vi "HdrLinePar.vi"(0 "String":string) -> (1 "Paramètre":string, 2 "Valeur":string, 3 "Commentaire":string)   [LabVIEW 2011]
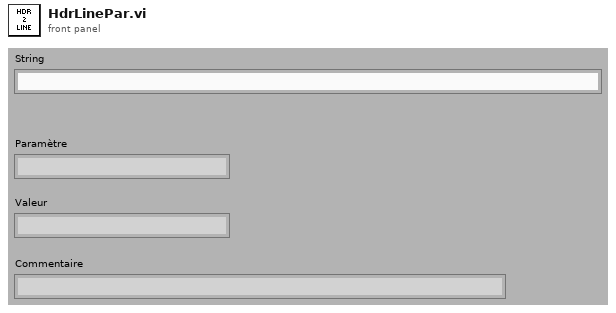
[diagram p1: front panel]
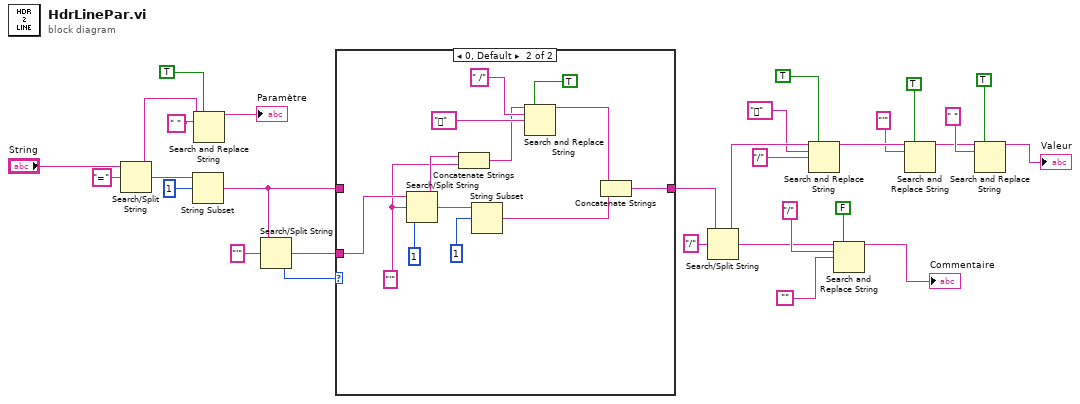
[diagram p0: block diagram]
diagram:
  n1 = Search/Split String(string="String", search string/char (-)="=") -> (substring before match=w25:string, match + rest of string=w27:string)  [unwired: 1 in, 1 out]
  n2 = String Subset(string=w27, offset (0)=1) -> (substring=w18:string)  [unwired: 1 in]
  n3 = Search and Replace String(replace all?=TRUE ("replace all? (F)"), input string=w25, search string=" ") -> (result string=→"Paramètre":string)  [unwired: 5 in, 3 out]
  n4 = Search/Split String(string=w18, search string/char (-)="'") -> (match + rest of string=w17:string, offset of match=w20:i32)  [unwired: 1 in, 1 out]
  n5 = case shown="0, Default" w20 {
    tunnel: [w31 w34] -> w19
    tunnel: w18 -> [w31 _]
    tunnel: w17 -> [_ w44]
    frame -1 {
    }
    frame 0, Default {
      w38 = "'" ("search string/char (-)")
      n6 = Search/Split String(string=w44, search string/char (-)=w38, offset (0)=1) -> (substring before match=w39:string, match + rest of string=w43:string)  [unwired: 1 out]
      n7 = Concatenate Strings(w39, w38) -> (w37:string)
      n8 = String Subset(string=w43, offset (0)=1) -> (substring=w35:string)  [unwired: 1 in]
      n9 = Search and Replace String(replace all?=TRUE ("replace all? (F)"), input string=w37, search string=" /", replace string="" ("search string")) -> (result string=w36:string)  [unwired: 4 in, 3 out]
      n10 = Concatenate Strings(w36, w35) -> (w34:string)
    }
  }
  n11 = Search/Split String(string=w19, search string/char (-)="/") -> (substring before match=w16:string, match + rest of string=w10:string)  [unwired: 1 in, 1 out]
  n12 = Search and Replace String(replace all?=TRUE ("replace all? (F)"), input string=w16, search string="", replace string="/" ("replace string (\"\")")) -> (result string=w7:string)  [unwired: 4 in, 3 out]
  n13 = Search and Replace String(replace all?=FALSE ("replace all? (F)"), input string=w10, search string="/", replace string="") -> (result string=→"Commentaire":string)  [unwired: 4 in, 3 out]
  n14 = Search and Replace String(replace all?=TRUE ("replace all? (F)"), input string=w7, search string="'" ("search string/char (-)")) -> (result string=w2:string)  [unwired: 5 in, 3 out]
  n15 = Search and Replace String(replace all?=TRUE ("replace all? (F)"), input string=w2, search string=" " ("search string/char (-)")) -> (result string=→"Valeur":string)  [unwired: 5 in, 3 out]
